vi "Bandgap.vi"() -> ()   [LabVIEW 2013]
uses:
  <vilib>/Utility/file.llb/Write To Spreadsheet File (DBL).vi
panel:
  in  "Path C:\\intlab bandgap\\file.xls":path
  out "?":dbl[](array[numeric]) format="%.2f"
  out "?":dbl format="%.2f"
  out "Ln(I) vs. V":cluster{dbl[], dbl[]}(graph)
  in  "?":bool
  in  "Data points":dbl=50.0
  in  "Resistance":dbl=10000.0
  out "Current\nthrough\njunction(mA)":dbl=-0.00027901785714285734 format="%.2e"
  out "Voltage\nacross\njunction(V)":dbl=-0.0048828125 format="%.3f"
  in  "Voltage\ncontrol":dbl step=0.05 format="%.2f"
  in  "?":bool
  # "Make sure the circuit is wired properly.  Channel 0 reads the voltage\nacross the junction.  Channel 1 reads the voltage across the resistor\nand uses the resistance input to calculate the current.  Read these \ninstructions and then scroll down to the inputs and the graph below to\ndo the experiment.\n(1)   Input your resistor value.  Should be about 10000 ohms.\n(2)   Input a file name.  Make sure it doesn't already exist, or else data\n           will be appended to it.\n(3)   Go to Operate>>Run and run the program.\n(4)   Adjust voltage control.  When \"Voltage across junction\" no longer\n           varies, press \"Take data point\".\n(5)   After finishing data collection for one temperature, press the\n          \"Temp. done\" button.  Your data is now written to the Excel file\n           in three columns  ==>  V, I, Ln(I)\n(6)   Go to Operate>>Reinitialize all to Default"
  # "E"
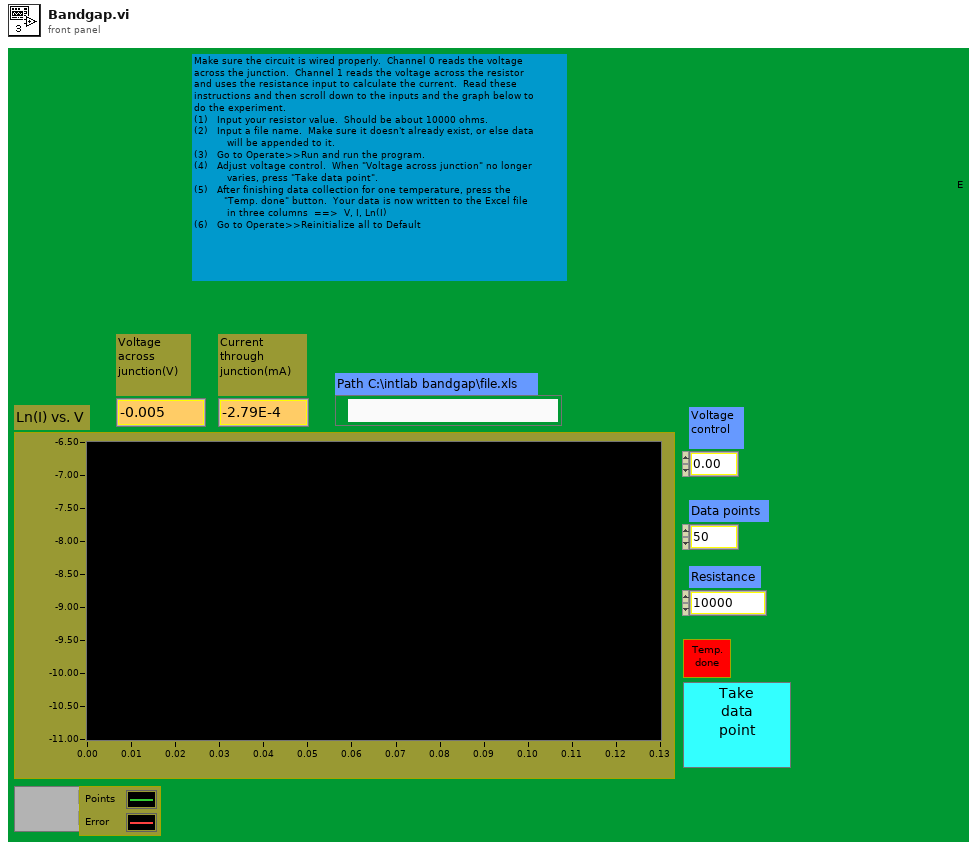
[diagram p1: front panel]
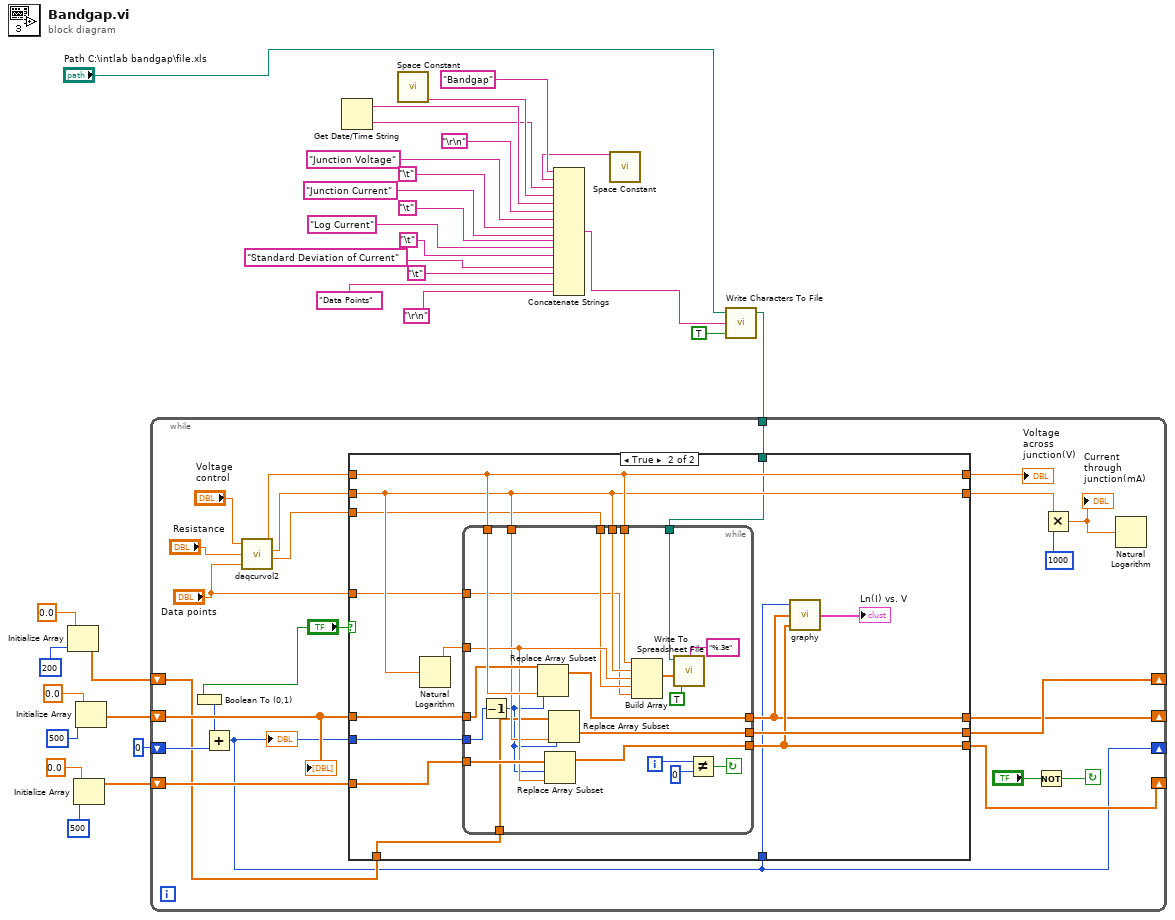
[diagram p0: block diagram]
diagram:
  n1 = Initialize Array(0.0, 200) -> (w21:dbl[])
  n2 = Initialize Array(0.0, 500) -> (w24:dbl[])
  n3 = Initialize Array(0.0, 500) -> (w25:dbl[])
  n4 = Get Date/Time String() -> (date string=w7:string, time string=w3:string)  [unwired: 3 out]
  n5 = call <vilib>:"Space Constant.vi"() -> ("String"=w4:string)
  n6 = call <vilib>:"Space Constant.vi"() -> ("String"=w5:string)
  n7 = Concatenate Strings("Bandgap" ("Spreadsheet Name"), w5, w3, w4, w7, "\r\n", "Junction Voltage", "\t", "Junction Current", "\t", "Log Current", "\t", "Standard Deviation of Current", "\t", "Data Points", "\r\n") -> (w19:string)
  n8 = call <vilib>:"Write Characters To File.vi"("append to file? (new file:F)"=TRUE, "character string"=w19, "file path (dialog if empty)"="Path C:\\intlab bandgap\\file.xls") -> ("new file path (Not A Path if cancelled)"=w1:path)  [unwired: 2 out]
  n9 = while {
    shift-left: w21 -> [w43]
    shift-right: [w42] -> _
    shift-left: w24 -> [w44]
    shift-right: [w41] -> _
    shift-left: w25 -> [w45]
    shift-right: [w40] -> _
    shift-left: 0 -> [w46]
    shift-right: [w39] -> _
    tunnel: w1 -> [w31]
    stop <- w47 continue-if-true
    n10 = Boolean To (0,1)(Boolean="?") -> (0, 1=w33:i16)
    n11 = Add(x=w33, y=w46) -> (x+y=w39:i32)
    "?" <- w39
    n12 = call "daqcurvol2.vi"("Voltage\ncontrol"="Voltage\ncontrol", "Resistance"="Resistance", "Data points"="Data points") -> ("Voltage\nacross\njunction"=w35:dbl, "Current\nthrough\njunction"=w36:dbl, "Current through\nStan Dev"=w34:dbl)  [unwired: 1 out]
    n13 = case shown="True" "?" {
      tunnel: [w58 w72] -> w50
      tunnel: w35 -> [w58 w72]
      tunnel: w36 -> [w57 w66]
      tunnel: [w57 w66] -> w49
      tunnel: w45 -> [w56 w71]
      tunnel: w39 -> [_ w70]
      tunnel: [w56 w61] -> w40
      tunnel: w44 -> [w55 w69]
      tunnel: [w55 w62] -> w41
      tunnel: w43 -> [w54 w68]
      tunnel: [w54 w67] -> w42
      tunnel: w39 -> [_ w60]
      tunnel: w34 -> [_ w63]
      tunnel: "Data points" -> [_ w65]
      tunnel: w31 -> [_ w64]
      frame False {
      }
      frame True {
        n14 = Natural Logarithm(1:w66) -> (0:w73:dbl)
        n15 = while {
          tunnel: [w81] -> w67
          tunnel: w68 -> [w82]
          tunnel: [w83] -> w62
          tunnel: w66 -> [w84]
          tunnel: w69 -> [w87]
          tunnel: [w89] -> w61
          tunnel: w70 -> [w88]
          tunnel: w71 -> [w86]
          tunnel: w72 -> [w90]
          tunnel: w72 -> [w91]
          tunnel: w66 -> [w93]
          tunnel: w73 -> [w85]
          tunnel: w63 -> [w77]
          tunnel: w65 -> [w76]
          tunnel: w64 -> [w74]
          i -> [w80]
          stop <- w78 continue-if-true
          n16 = Decrement(x=w88) -> (x-1=w75:i32)
          n17 = Replace Array Subset(array=w86, new element=w90, index=w75) -> (w89:dbl[])
          n18 = Replace Array Subset(array=w87, new element=w85, index=w75) -> (w83:dbl[])
          n19 = Replace Array Subset(array=w82, new element=w84, index=w75) -> (w81:dbl[])
          n20 = Build Array(w91, w93, w85, w77, w76) -> (w92:dbl[])
          n21 = call-poly <vilib>:"Write To Spreadsheet File.vi"("format (%.3f)"="%.3e", "append to file? (new file:F)"=TRUE, "1D data"=w92, "file path (dialog if empty)"=w74) -> ()  [unwired: 2 in, 3 out]
          n22 = Not Equal?(x=w80, y=0) -> (x != y?=w78:bool)
        }
        n23 = call "graphy.vi"("Y array"=w62, "X array"=w61, "Elements"=w60) -> (0:→"Ln(I) vs. V":cluster{dbl[], dbl[]})
      }
    }
    "Voltage\nacross\njunction(V)" <- w50
    n24 = Not(x="?") -> (.not. x?=w47:bool)
    n25 = Multiply(x=w49, y=1000) -> (x*y=w51:dbl)
    "Current\nthrough\njunction(mA)" <- w51
    n26 = Natural Logarithm(1:w51) -> ()  [unwired: 1 out]
    "?" <- w45
  }
